vi "Entry Display Module.vi"(8 "error in":errorcluster) -> (0 "error out":errorcluster)   [LabVIEW 2018, in "Entry Console.lvlib"]
doc: "This is the top level of the entry console module (a free running module of the Car WAsh simulator). \n\nIt is closed using a user event. It communicates with the other modules using a queue based API which has comms modules that can be swapped if required."
uses:
  Entry Console.lvlib
  Private Controls/Module Action.ctl
  Private Controls/Module Data Cluster.ctl
  Public Controls/Entry Console.ctl
panel:
  in  "Entry GUI":T1
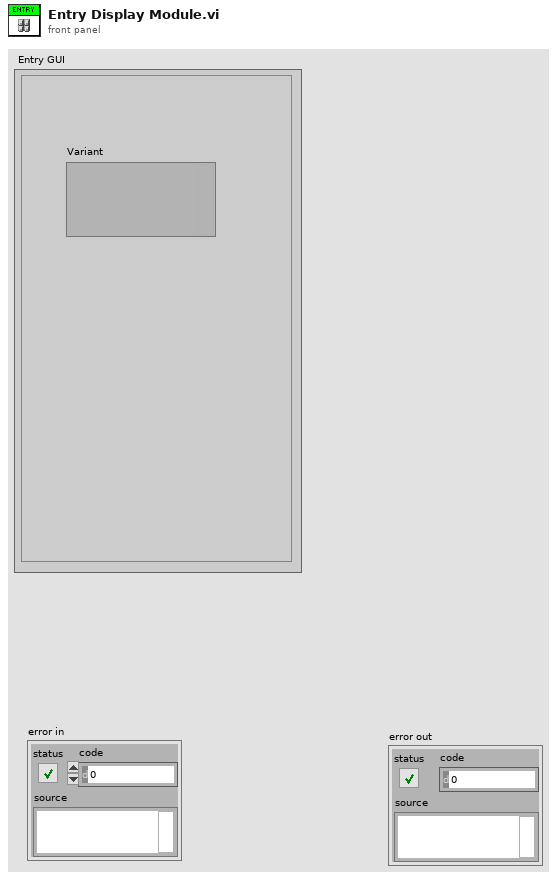
[diagram p1: front panel]
types:
  T1 = typedef "Entry Console.lvlib/Entry Console.ctl" = cluster{"Variant":variant}
  T2 = typedef "Entry Console.lvlib/Module Data Cluster.ctl" = cluster{"Variant":variant, "action":T3}
  T3 = typedef "Entry Console.lvlib/Module Action.ctl" = enum16{"error", "exit", "Start Wash", "init", "Enable Wash Buttons"}
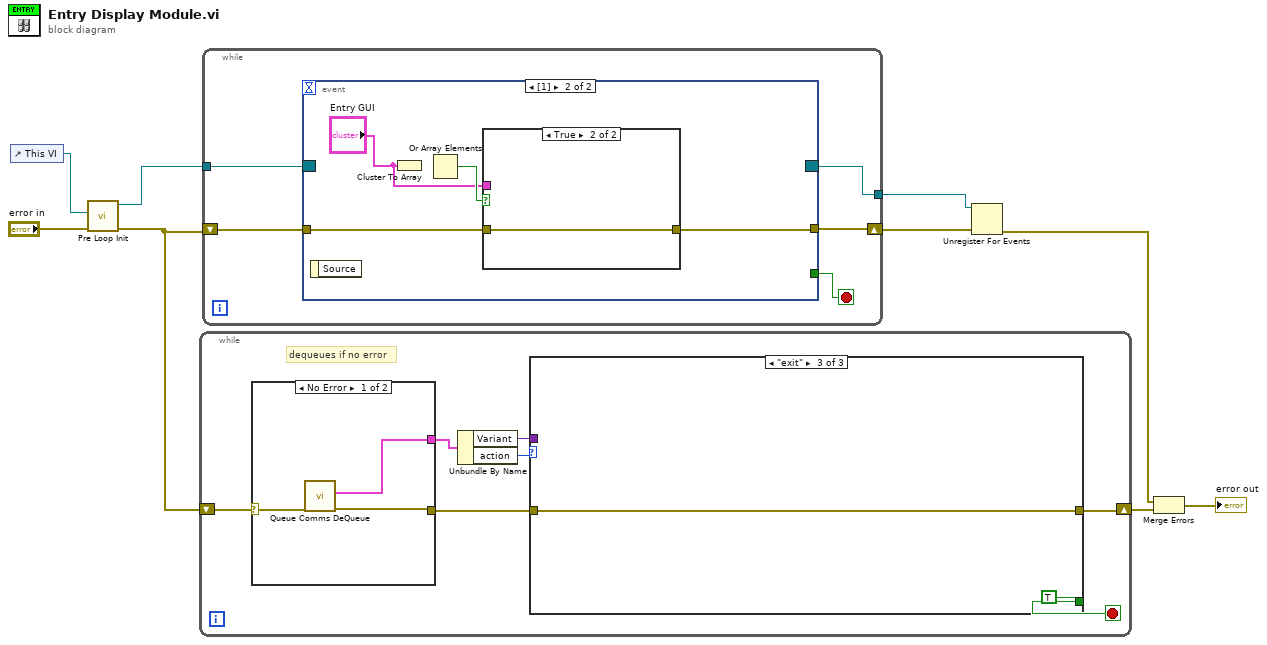
[diagram p0: block diagram]
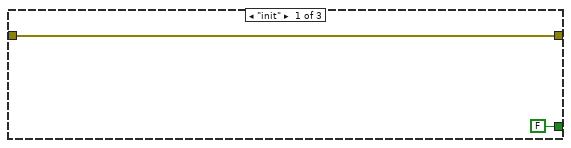
[diagram p2: hidden frame]
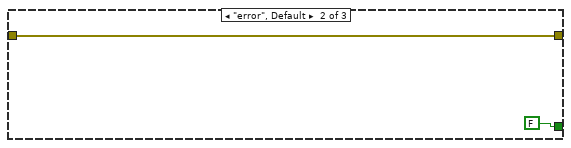
[diagram p3: hidden frame]
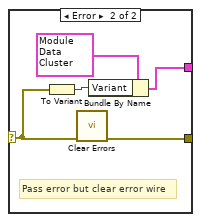
[diagram p4: hidden frame]
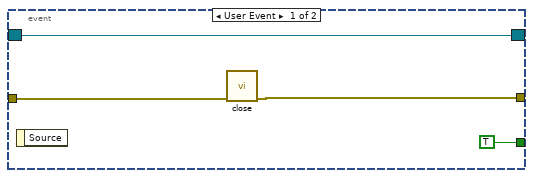
[diagram p5: hidden frame]
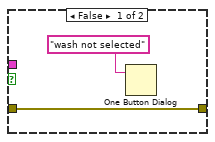
[diagram p6: hidden frame]
diagram:
  n1 = control-ref of="This VI"() -> (w9:refnum<vi>)
  n2 = call "Pre Loop Init.vi"("error in"="error in", "Ref In"=w9) -> ("error out"=w6:errorcluster, "Event Registration Refnum"=w8:refnum<event-registration>)  [unwired: 8 in]
  n3 = while {
    shift-right: [w12] -> w3
    shift-left: w6 -> [w16]
    stop <- w10 stop-if-true
    # "dequeues if no error"
    n4 = case shown="No Error" w16 {
      selector: w16 -> [w25 w30]
      tunnel: [w24 w26] -> w15
      tunnel: [w23 w29] -> w11
      frame No Error {
        n5 = call "Queue Comms DeQueue.vi"("error in"=w25) -> ("error out"=w23:errorcluster, "element"=w24:T2)  [unwired: 9 in]
      }
      frame Error {
        # "Pass error but clear error wire"
        n6 = To Variant(anything=w30) -> (Variant=w27:variant)
        n7 = call <vilib>:"Clear Errors.vi"("error in (no error)"=w30) -> ("error out"=w29:errorcluster)  [unwired: 5 in, 1 out]
        n8 = Bundle By Name(cluster=T2 {"Variant"=variant, "action"=enum."error"} ("element"), "Variant"=w27) -> (w26:T2)
      }
    }
    n9 = Unbundle By Name(w15) -> ("Variant"=w13:variant, "action"=w14:T3)
    n10 = case shown="\"exit\"" w14 {
      tunnel: w13 -> [_ _ _]
      tunnel: [w18 w20 w22] -> w12
      tunnel: w11 -> [w18 w20 w22]
      tunnel: [FALSE FALSE TRUE] -> w10
      frame "init" {
      }
      frame "error", Default {
      }
      frame "exit" {
      }
    }
  }
  n11 = while {
    shift-right: [w34] -> w5
    shift-left: w6 -> [w35]
    tunnel: w8 -> [w33]
    tunnel: [w31] -> w4
    stop <- w32 stop-if-true
    n12 = event shown="[1]" {
      selector: w33 -> [w36 _]
      dyn-events: [w36 _] -> w31
      timeout: _ -> [_ _]
      tunnel: w35 -> [w39 w43]
      tunnel: [w38 w41] -> w34
      tunnel: [TRUE _] -> w32
      event User Event {
        n13 = event-data() -> ()  [unwired: 1 in, 1 out]
        n14 = call "close.vi"("error in"=w39) -> ("error out"=w38:errorcluster)  [unwired: 10 in]
      }
      event #1 (no event record) {
        n15 = event-data() -> ()  [unwired: 1 in, 1 out]
        n16 = Cluster To Array(cluster="Entry GUI") -> ()  [unwired: 1 out]
        n17 = Or Array Elements() -> (logical OR=w42:bool)  [unwired: 1 in]
        n18 = case shown="True" w42 {
          tunnel: w43 -> [w44 w46]
          tunnel: "Entry GUI" -> [_ _]
          tunnel: [w44 w46] -> w41
          frame False {
            n19 = One Button Dialog(message="wash not selected") -> ()  [unwired: 1 in, 1 out]
          }
          frame True {
          }
        }
      }
    }
  }
  n20 = Unregister For Events(event registration refnum=w4, error in=w5) -> (error out=w1:errorcluster)
  n21 = Merge Errors(w1, w3) -> (→"error out":errorcluster)
